vi "AddNewLog.vi"(8 "error in":errorcluster, 9 "Details":string, 10 "General Info":string, 11 "Logging file refnum in":refnum<file>) -> (0 "error out":errorcluster, 3 "Logging file refnum out":refnum<file>)   [LabVIEW 2019]
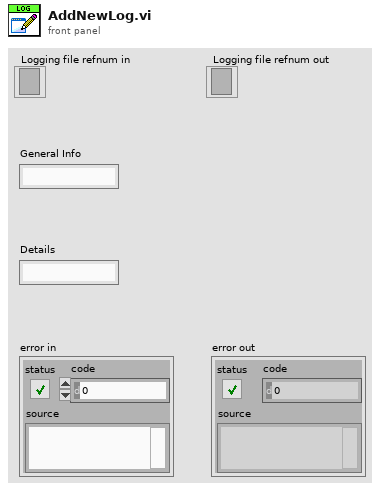
[diagram p1: front panel]
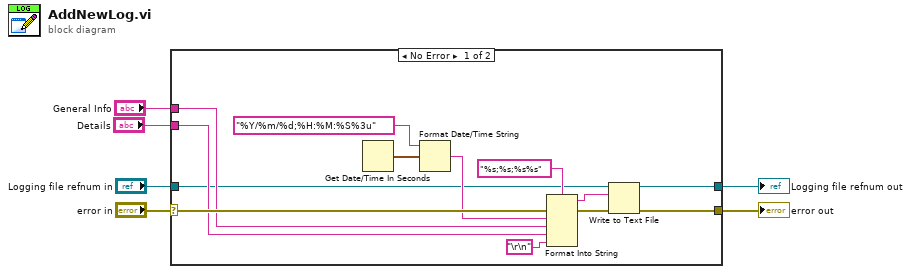
[diagram p0: block diagram]
diagram:
  n1 = case shown="No Error" "error in" {
    selector: "error in" -> [w18 w21]
    tunnel: [w19 w21] -> w5
    tunnel: "General Info" -> [w14 _]
    tunnel: "Details" -> [w15 _]
    tunnel: "Logging file refnum in" -> [w9 w20]
    tunnel: [w8 w20] -> w1
    frame No Error {
      n2 = Get Date/Time In Seconds() -> (seconds since 1Jan1904=w12:timestamp)
      n3 = Format Date/Time String(time format string (%c)="%Y/%m/%d;%H:%M:%S%3u", seconds (now)=w12) -> (date/time string=w11:string)  [unwired: 1 in]
      n4 = Format Into String(format string="%s;%s;%s%s", error in=w18, w11, w14, w15, "\r\n") -> (resulting string=w10:string, error out=w17:errorcluster)  [unwired: 1 in]
      n5 = Write to Text File(file (use dialog)=w9, text=w10, error in=w17) -> (refnum out=w8:refnum<file>, error out=w19:errorcluster)  [unwired: 1 in, 1 out]
    }
    frame Error {
    }
  }
  "error out" <- w5
  "Logging file refnum out" <- w1
